vi "load parameters.vi"() -> (2 "parameters":T13 {"messageHandler"."params"."controlChannels"."ballControl" items=["Module6/output0", "Module6/output1", "Module6/output2", "Module6/output3", "Not-Used"]; "messageHandler"."params"."controlChannels"."butterflyControl" items=["Module6/output0", "Module6/output1", "Module6/output2", "Module6/output3", "Not-Used"]; "messageHandler"."params"."controlChannels"."speedControl" items=["Module6/output0", "Module6/output1", "Module6/output2", "Module6/output3", "Not-Used"]})   [LabVIEW 2018]
uses:
  type defs/message handler data.ctl
  customVI/liveData/state.ctl
  type defs/comms loop data.ctl
  Github/ICL-LabVIEW_General/Incident logger/Incident logger.lvclass
  <vilib>/Modbus/master/Modbus Master.lvclass
  type defs/data stream data.ctl
  type defs/data processor data.ctl
  type defs/channelLimitControl.ctl
  type defs/limitActions.ctl
  type defs/file IO data.ctl
  type defs/channelControl.ctl
  RT/Type Defs/channelScalingTypes.ctl
  RT/Type Defs/scalingMethods.ctl
  Github/ICL-LabVIEW_General/data channels/parent class/Data Channel.lvclass
  type defs/UI loop data.ctl
  type defs/error messages data.ctl
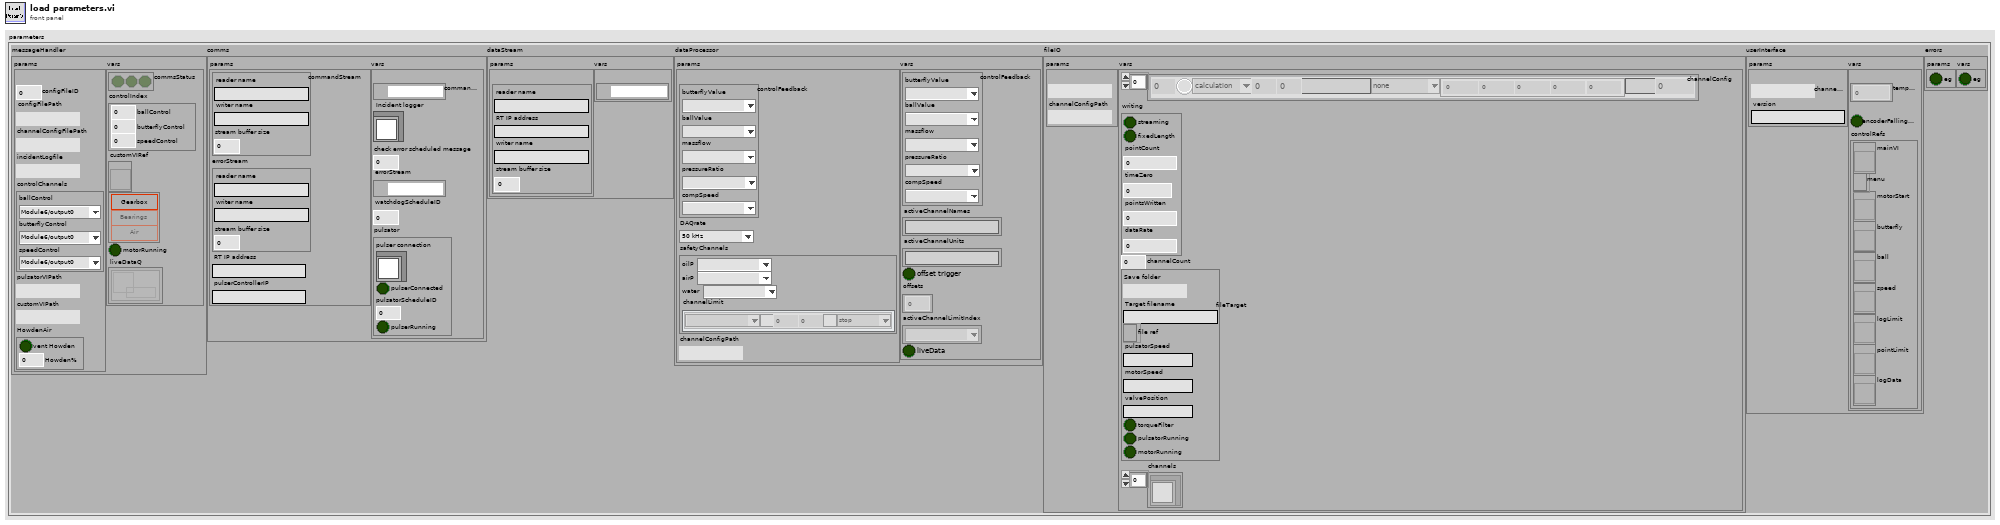
[diagram p1: front panel]
types:
  T1 = typedef "message handler data.ctl" = cluster{"params":cluster{"configFileID":u32, "configFilePath":path, "channelConfigFilePath":path, "incidentLogfile":path, "controlChannels":cluster{"ballControl":u16, "butterflyControl":u16, "speedControl":u16}, "pulsatorVIPath":path, "customVIPath":path, "HowdenAir":cluster{"vent Howden":bool, "Howden%":dbl}}, "vars":cluster{"commsStatus":bool[], "controlIndex":cluster{"ballControl":u16, "butterflyControl":u16, "speedControl":u16}, "customVIRef":refnum<vi>, "Interlocks":cluster{"gearboxOil":bool, "bearingOil":bool, "gearboxAir":bool}, "motorRunning":bool, "liveDataQ":refnum<queue>[]}}
  T2 = typedef "comms loop data.ctl" = cluster{"params":cluster{"commandStream":cluster{"reader name":string, "writer name":string, "stream buffer size":i32}, "errorStream":cluster{"reader name":string, "writer name":string, "stream buffer size":i32}, "RT IP address":string, "pulserControllerIP":string}, "vars":cluster{"commandStream":refnum<k21>, "Incident logger":refnum<class "Incident logger.lvclass">, "check error scheduled message":u32, "errorStream":refnum<k21>, "watchdogScheduleID":u32, "pulsator":cluster{"pulser connection":refnum<class "Modbus Master.lvclass">, "pulserConnected":bool, "pulsatorScheduleID":u32, "pulserRunning":bool}}}
  T3 = typedef "data stream data.ctl" = cluster{"params":cluster{"Stream":cluster{"reader name":string, "RT IP address":string, "writer name":string, "stream buffer size":i32}}, "vars":cluster{"data stream":refnum<k21>}}
  T4 = typedef "data processor data.ctl" = cluster{"params":cluster{"controlFeedback":cluster{"butterflyValue":u16, "ballValue":u16, "massflow":u16, "pressureRatio":u16, "compSpeed":u16}, "DAQrate":enum16{"50 kHz", "25 kHz", "16.6 kHz", "12.5 kHz", "10 kHz", "8.33 kHz", "7.14 kHz", "6.25 kHz", "5.55 kHz", "5 kHz"}, "safetyChannels":cluster{"oilP":u16, "airP":u16, "water":u16, "channelLimit":T5[]}, "channelConfigPath":path}, "vars":cluster{"controlFeedback":cluster{"butterflyValue":u16, "ballValue":u16, "massflow":u16, "pressureRatio":u16, "compSpeed":u16}, "activeChannelNames":string[], "activeChannelUnits":string[], "offset trigger":bool, "offsets":dbl[], "activeChannelLimitIndex":u16[], "liveData":bool}}
  T5 = typedef "channelLimitControl.ctl" = cluster{"channelID":u16, "Enabled":bool, "warnValue":dbl, "limitValue":dbl, "Invert":bool, "limitAction":T6}
  T6 = typedef "limitActions.ctl" = enum16{"stop", "shutdown", "ignore"}
  T7 = typedef "file IO data.ctl" = cluster{"params":cluster{"startFolder":path, "channelConfigPath":path}, "vars":cluster{"channelConfig ":T8[], "writing":cluster{"streaming":bool, "fixedLength":bool, "pointCount":u32, "timeZero":dbl, "pointsWritten":u32, "dataRate":u16}, "channelCount":u16, "fileTarget":cluster{"Save folder":path, "Target filename":string, "file ref":refnum<file>, "pulsatorSpeed":string, "motorSpeed":string, "valvePosition":string, "torqueFilter":bool, "pulsatorRunning":bool, "motorRunning":bool}, "channels":refnum<class "Data Channel.lvclass">[]}}
  T8 = typedef "channelControl.ctl" = cluster{"index":u16, "active":bool, "channelType":T9, "module":u16, "terminal":u16, "channelName":string, "scalingMethod":T10, "scalingParameters":dbl[], "scaledUnits":string, "tempOffset":dbl}
  T9 = typedef "channelScalingTypes.ctl" = enum16{"calculation", "measurement", "scanivalve", "output", "digital"}
  T10 = typedef "scalingMethods.ctl" = enum16{"none", "linear", "thermocouple", "polynomial", "encoder", "RTD"}
  T11 = typedef "UI loop data.ctl" = cluster{"params":cluster{"channelConfigPath":path, "version":string}, "vars":cluster{"tempOffsets":dbl[], "encoderFallingEdge":bool, "controlRefs":cluster{"mainVI":refnum<vi>, "menu":refnum<k9>, "motorStart":refnum<vi>, "butterfly":refnum<vi>, "ball":refnum<vi>, "speed":refnum<vi>, "logLimit":refnum<vi>, "pointLimit":refnum<vi>, "logData":refnum<vi>}}}
  T12 = typedef "error messages data.ctl" = cluster{"params":cluster{"eg":bool}, "vars":cluster{"eg":bool}}
  T13 = cluster{"messageHandler":T1, "comms":T2, "dataStream":T3, "dataProcessor":T4, "fileIO":T7, "userInterface":T11, "errors":T12}
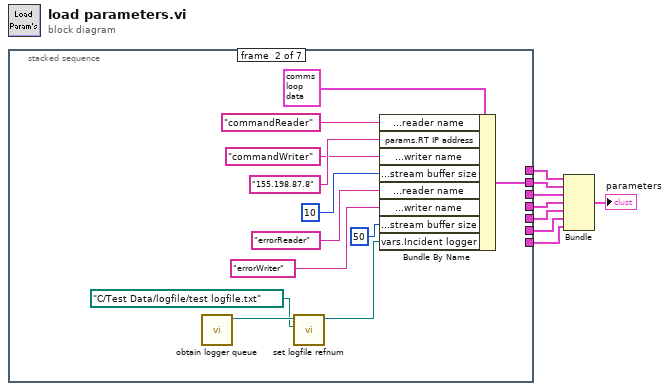
[diagram p0: block diagram]
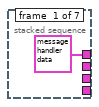
[diagram p2: hidden frame]
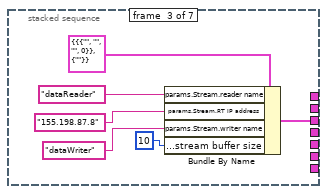
[diagram p3: hidden frame]
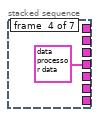
[diagram p4: hidden frame]
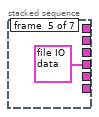
[diagram p5: hidden frame]
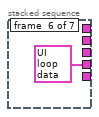
[diagram p6: hidden frame]
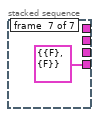
[diagram p7: hidden frame]
diagram:
  n1 = stacked-sequence {
    tunnel: [T1 {"params"={"configFileID"=0, "configFilePath"=path "", "channelConfigFilePath"=path "", "incidentLogfile"=path "", "controlChannels"={"ballControl"=0, "butterflyControl"=0, "speedControl"=0}, "pulsatorVIPath"=path "", "customVIPath"=path "", "HowdenAir"={"vent Howden"=FALSE, "Howden%"=0.0}}, "vars"={"commsStatus"=[], "controlIndex"={"ballControl"=0, "butterflyControl"=0, "speedControl"=0}, "customVIRef"=refnum, "Interlocks"={"gearboxOil"=FALSE, "bearingOil"=FALSE, "gearboxAir"=FALSE}, "motorRunning"=FALSE, "liveDataQ"=[]}} ("messageHandler") _ _ _ _ _ _] -> w8
    tunnel: [_ w20 _ _ _ _ _] -> w7
    tunnel: [_ _ _ _ _ T11 {"params"={"channelConfigPath"=path "", "version"=""}, "vars"={"tempOffsets"=[], "encoderFallingEdge"=FALSE, "controlRefs"={"mainVI"=refnum, "menu"=refnum, "motorStart"=refnum, "butterfly"=refnum, "ball"=refnum, "speed"=refnum, "logLimit"=refnum, "pointLimit"=refnum, "logData"=refnum}}} ("userInterface") _] -> w6
    tunnel: [_ _ w26 _ _ _ _] -> w5
    tunnel: [_ _ _ T4 {"params"={"controlFeedback"={"butterflyValue"=0, "ballValue"=0, "massflow"=0, "pressureRatio"=0, "compSpeed"=0}, "DAQrate"=enum."50 kHz", "safetyChannels"={"oilP"=0, "airP"=0, "water"=0, "channelLimit"=[]}, "channelConfigPath"=path ""}, "vars"={"controlFeedback"={"butterflyValue"=0, "ballValue"=0, "massflow"=0, "pressureRatio"=0, "compSpeed"=0}, "activeChannelNames"=[], "activeChannelUnits"=[], "offset trigger"=FALSE, "offsets"=[], "activeChannelLimitIndex"=[], "liveData"=FALSE}} ("dataProcessor") _ _ _] -> w4
    tunnel: [_ _ _ _ T7 {"params"={"startFolder"=path "", "channelConfigPath"=path ""}, "vars"={"channelConfig "=[], "writing"={"streaming"=FALSE, "fixedLength"=FALSE, "pointCount"=0, "timeZero"=0.0, "pointsWritten"=0, "dataRate"=0}, "channelCount"=0, "fileTarget"={"Save folder"=path "", "Target filename"="", "file ref"=refnum, "pulsatorSpeed"="", "motorSpeed"="", "valvePosition"="", "torqueFilter"=FALSE, "pulsatorRunning"=FALSE, "motorRunning"=FALSE}, "channels"=[]}} ("fileIO") _ _] -> w3
    tunnel: [_ _ _ _ _ _ T12 {"params"={"eg"=FALSE}, "vars"={"eg"=FALSE}} ("errors")] -> w2
    frame #0 {
    }
    frame #1 {
      n2 = call "obtain logger queue.vi"() -> ("Incident logger out"=w13:refnum<class "Incident logger.lvclass">)  [unwired: 10 in, 1 out]
      n3 = call "set logfile refnum.vi"("Logfile"=path "C:/Test Data/logfile/test logfile.txt", "Incident logger in"=w13) -> ("Incident logger out"=w11:refnum<class "Incident logger.lvclass">)  [unwired: 8 in, 1 out]
      n4 = Bundle By Name(cluster=T2 {"params"={"commandStream"={"reader name"="", "writer name"="", "stream buffer size"=0}, "errorStream"={"reader name"="", "writer name"="", "stream buffer size"=0}, "RT IP address"="", "pulserControllerIP"=""}, "vars"={"commandStream"="", "Incident logger"=refnum, "check error scheduled message"=0, "errorStream"="", "watchdogScheduleID"=0, "pulsator"={"pulser connection"=refnum, "pulserConnected"=FALSE, "pulsatorScheduleID"=0, "pulserRunning"=FALSE}}} ("comms"), "params.commandStream.reader name"="commandReader", "params.RT IP address"="155.198.87.8" ("params.commandStream.RT IP address"), "params.commandStream.writer name"="commandWriter", "params.commandStream.stream buffer size"=10, "params.errorStream.reader name"="errorReader", "params.errorStream.writer name"="errorWriter", "params.errorStream.stream buffer size"=50, "vars.Incident logger"=w11) -> (w20:T2)
    }
    frame #2 {
      n5 = Bundle By Name(cluster=T3 {"params"={"Stream"={"reader name"="", "RT IP address"="", "writer name"="", "stream buffer size"=0}}, "vars"={"data stream"=""}} ("dataStream"), "params.Stream.reader name"="dataReader", "params.Stream.RT IP address"="155.198.87.8", "params.Stream.writer name"="dataWriter", "params.Stream.stream buffer size"=10) -> (w26:T3)
    }
    frame #3 {
    }
    frame #4 {
    }
    frame #5 {
    }
    frame #6 {
    }
  }
  n6 = Bundle("messageHandler"=w8, "comms"=w7, "dataStream"=w5, "dataProcessor"=w4, "fileIO"=w3, "userInterface"=w6, "errors"=w2) -> (→"parameters":T13)  [unwired: 1 in]
